vi "Initialize_GL.vi"(0 "Motion Settings":T1={"No Motion?"=FALSE, "Motion System"=enum."NI 735x", "Motion Bd ID"=1, "Motion Profile"="SMAC1", "# Axis"=1, "Reverse Z axis?"=TRUE, "SMAC Axis"=0, "scan pair"=enum."y-(x) scan", "RT fps"=6.0, "Steps per mm"=[1000, 1000, 1000, 1000], "Motor Parameters"={"velocity ct/s"=[10000.0, 10000.0, 10000.0, 50000.0], "accel ct/s^2"=[50000.0, 50000.0, 50000.0, 200000.0]}, "One Way Scan"=FALSE, "Reverse One Way Scan"=FALSE, "Global Position (mm)"=[], "Plane"=0, "Distance between\nscan lines (um)"=0.0, "Distance between\nscan planes (um)"=0.0, "number of scan planes"=1, "Total steps in line"=0, "Xtra plane\ndistance  (um)"=100, "Xtra planes "=1, "Add Axis"=FALSE, "overshoot cts"=200, "BKPT Shift"=0, "Scan Start Time (ms)"=0, "ESP VISA"="GPIB::1::INSTR", "3rd Axis"=1, "GL Ref Out"=refnum, "Galil Address"=""} {"3rd Axis" items=["x", "y", "z", "w"]; "Xtra planes" min=1; "Xtra plane\ndistance  (um)" min=0; "Distance between\nscan planes (um)" format="%.2f"; "Distance between\nscan lines (um)" format="%.2f"; "SMAC Axis" items=["None"=0, "Axis 1"=1, "Axis 2"=2, "Axis 3"=3, "Axis 4"=4, "Axis 5"=5, "Axis 6"=6, "Axis 7"=7, "Axis 8"=8, "Vector Space 1"=17, "Vector Space 2"=18, "Vector Space 3"=19, "Vector Space 4"=20]; "Motion Bd ID" min=1 max=32 step=1}, 2 "Location":T5, 3 "error in":errorcluster) -> (5 "Motion Settings":T1={"No Motion?"=FALSE, "Motion System"=enum."NI 735x", "Motion Bd ID"=1, "Motion Profile"="SMAC1", "# Axis"=1, "Reverse Z axis?"=TRUE, "SMAC Axis"=0, "scan pair"=enum."y-(x) scan", "RT fps"=6.0, "Steps per mm"=[1000, 1000, 1000, 1000], "Motor Parameters"={"velocity ct/s"=[10000.0, 10000.0, 10000.0, 50000.0], "accel ct/s^2"=[50000.0, 50000.0, 50000.0, 200000.0]}, "One Way Scan"=FALSE, "Reverse One Way Scan"=FALSE, "Global Position (mm)"=[], "Plane"=0, "Distance between\nscan lines (um)"=0.0, "Distance between\nscan planes (um)"=0.0, "number of scan planes"=1, "Total steps in line"=0, "Xtra plane\ndistance  (um)"=100, "Xtra planes "=1, "Add Axis"=FALSE, "overshoot cts"=200, "BKPT Shift"=0, "Scan Start Time (ms)"=0, "ESP VISA"="GPIB::1::INSTR", "3rd Axis"=1, "GL Ref Out"=refnum, "Galil Address"=""} {"3rd Axis" items=["x", "y", "z", "w"]; "Xtra planes" min=1; "Xtra plane\ndistance  (um)" min=0; "Distance between\nscan planes (um)" format="%.2f"; "Distance between\nscan lines (um)" format="%.2f"; "SMAC Axis" items=["None"=0, "Axis 1"=1, "Axis 2"=2, "Axis 3"=3, "Axis 4"=4, "Axis 5"=5, "Axis 6"=6, "Axis 7"=7, "Axis 8"=8, "Vector Space 1"=17, "Vector Space 2"=18, "Vector Space 3"=19, "Vector Space 4"=20]; "Motion Bd ID" min=1 max=32 step=1}, 6 "Initialization Failed!!":bool, 7 "error out":errorcluster)   [LabVIEW 2022 SP3]
uses:
  NI_controller/-NI_MotionRoutines/MotionParameters.ctl
  NI_controller/-NI_MotionRoutines/MotionSys.ctl
  -MotionRoutines/ScanAxis.ctl
  -MotionRoutines/3rdAxis.ctl
  -ScanSystem/Controls/location.ctl
  Command Menu.ctl
  GL Axis Control.ctl
panel:
  # "1-D and 2-D B scan settings"
  # "1-D and 2-D B scan settings"
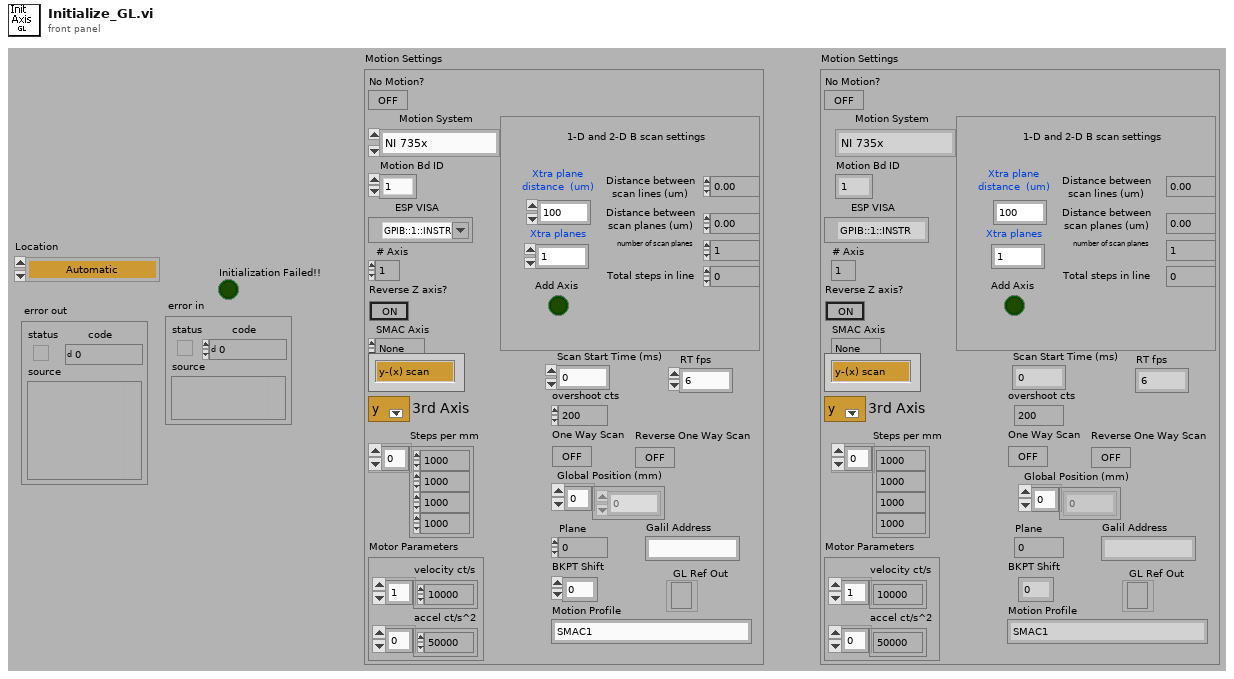
[diagram p1: front panel]
types:
  T1 = typedef "MotionParameters.ctl" = cluster{"No Motion?":bool, "Motion System":T2, "Motion Bd ID":u8, "Motion Profile":string, "# Axis":i8, "Reverse Z axis?":bool, "SMAC Axis":u16, "scan pair":T3, "RT fps":sgl, "Steps per mm":i32[], "Motor Parameters":cluster{"velocity ct/s":dbl[], "accel ct/s^2":dbl[]}, "One Way Scan":bool, "Reverse One Way Scan":bool, "Global Position (mm)":dbl[], "Plane":i32, "Distance between\nscan lines (um)":sgl, "Distance between\nscan planes (um)":sgl, "number of scan planes":i32, "Total steps in line":i32, "Xtra plane\ndistance  (um)":i32, "Xtra planes ":i32, "Add Axis":bool, "overshoot cts":i32, "BKPT Shift":i32, "Scan Start Time (ms)":u32, "ESP VISA":refnum<visa-resource-name>, "3rd Axis":T4, "GL Ref Out":refnum<k7>, "Galil Address":string}
  T2 = typedef "MotionSys.ctl" = enum16{"MM3000", "NI 735x", "Newport ESP", "No Motion Card", "Galil"}
  T3 = typedef "ScanAxis.ctl" = enum16{"y-(x) scan", "x-(y) scan", "z-(x) scan", "z-(y) scan", "y-(z) scan", "x-(z) scan", "w-(x) scan", "w-(y) scan", "w-(z) scan", "x-(w) scan", "y-(w) scan", "z-(w) scan"}
  T4 = typedef "3rdAxis.ctl" = u16
  T5 = typedef "location.ctl" = enum16{"Automatic", "WCM Main", "Hawaii", "Columbia MM3000", "Columbia  NI System", "NYU", "RRI 2", "UHI Allen", "CUMC RT", "Chiba", "Stony Brook", "WCM Microscopy", "WCM Aeoretch", "WCM Optics Lab", "WCM Main 2Axis", "WCM Rotation", "WCM SAM SMAC", "SERI GP", "SERI SAM 2023"}
  T6 = enum16{"Left Button", "Center Button", "Right Button", "Window Close"}
  T7 = typedef "Command Menu.ctl" = enum16{"CommandPassThrough", "Abort Motion", "Define Pos", "Velocity", "Acceleration", "Deceleration", "Position Rel", "Postion Abs", "Begin Move", "After Move", "Home", "KI", "KD", "KP", "IL", "Config I/O", "Set Bit", "Clear Bit", "Motor Off", "Moto On", "Status", "Execute", "Halt Execute", "HX Status", "Tell Velocity", "Check Motion", "BreakPoint", "Tell Position", "Current Code Line", "Tell Switches", "OC Force On", "OC Off", "Pos Soft Limit", "Rev Soft Limit"}
  T8 = cluster{"KD":i32, "KI":dbl, "KP":i32, "IL":i32}[]
  T9 = cluster{"KD":i32, "KI":i32, "KP":i32, "IL":i32}[]
  T10 = typedef "GL Axis Control.ctl" = u16
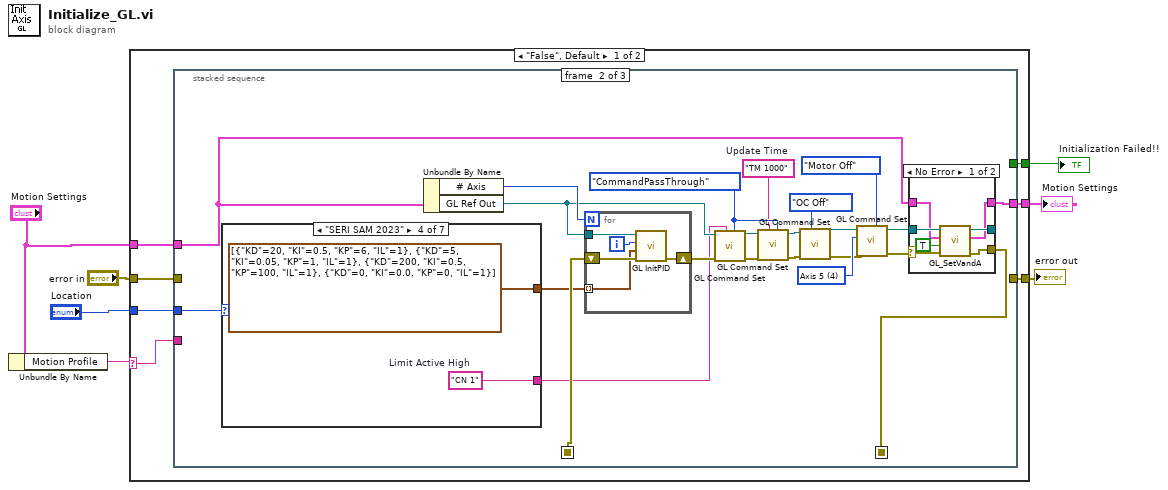
[diagram p0: block diagram]
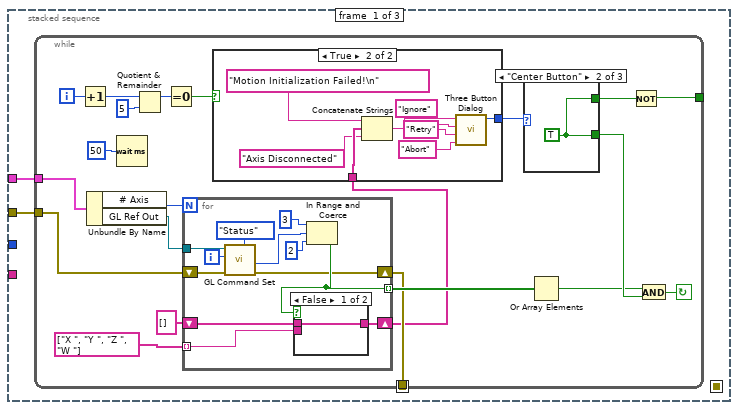
[diagram p2: hidden frame]
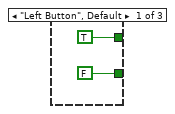
[diagram p3: hidden frame]
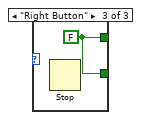
[diagram p4: hidden frame]
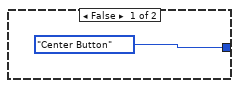
[diagram p5: hidden frame]
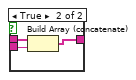
[diagram p6: hidden frame]
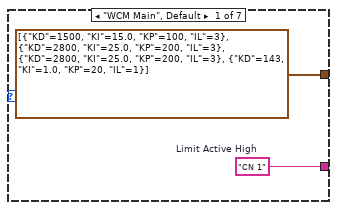
[diagram p8: hidden frame]
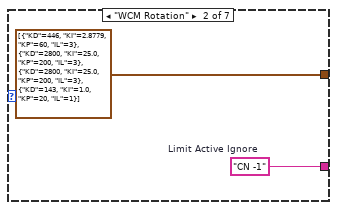
[diagram p9: hidden frame]
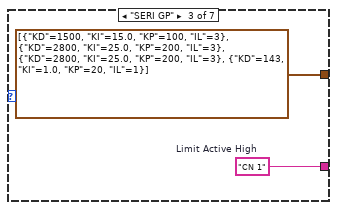
[diagram p10: hidden frame]
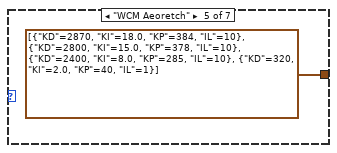
[diagram p11: hidden frame]
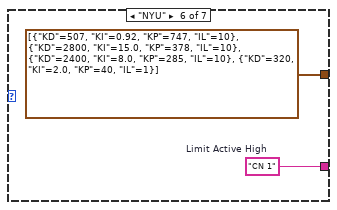
[diagram p12: hidden frame]
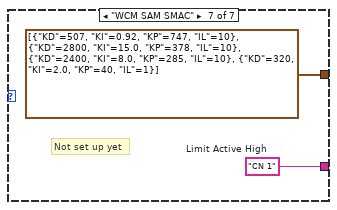
[diagram p13: hidden frame]
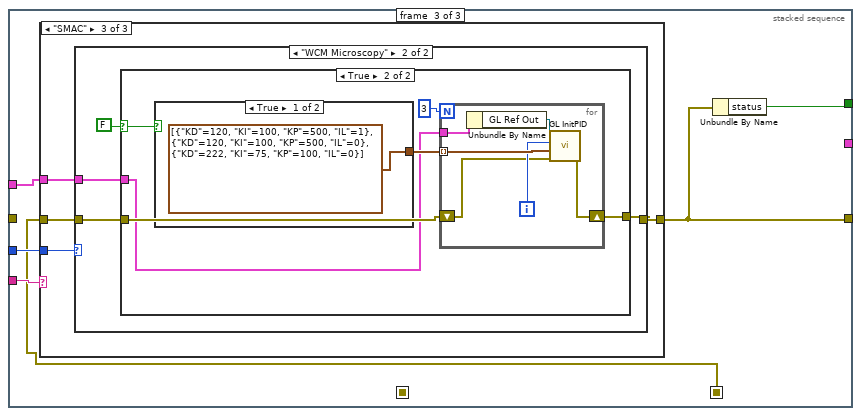
[diagram p14: hidden frame]
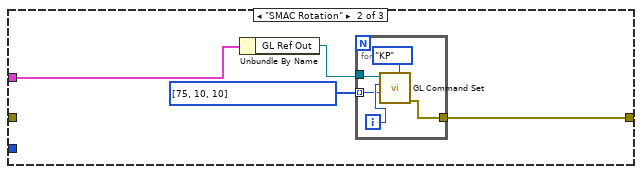
[diagram p16: hidden frame]
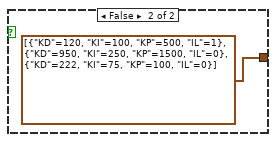
[diagram p19: hidden frame]
diagram:
  n1 = Unbundle By Name("Motion Settings") -> ("Motion Profile"=w4:string)
  n2 = case shown="\"False\", Default" w4 {
    selector: w4 -> [w11 _]
    tunnel: [w14 w160] -> w5
    tunnel: "Motion Settings" -> [w13 w159]
    tunnel: "error in" -> [w9 w160]
    tunnel: [w12 _] -> w6
    tunnel: "Location" -> [w10 _]
    tunnel: [w8 w159] -> w1
    frame "False", Default {
      n3 = stacked-sequence {
        seq-local: [w16 _ _] -> [_ w89 _]
        seq-local: [_ w69 _] -> [_ _ w121]
        tunnel: [_ _ w119] -> w14
        tunnel: w13 -> [w17 w87 w122]
        tunnel: w9 -> [w15 _ _]
        tunnel: [_ _ w120] -> w12
        tunnel: w11 -> [_ _ w124]
        tunnel: w10 -> [_ w68 w123]
        tunnel: [_ w70 _] -> w8
        frame #0 {
          n4 = while {
            tunnel: [w32] -> _
            tunnel: w17 -> [w25]
            tunnel: [w20] -> w16
            tunnel: w15 -> [w19]
            i -> [w36]
            stop <- w33 continue-if-true
            n5 = Increment(x=w36) -> (x+1=w34:i32)
            n6 = Unbundle By Name(w25) -> ("# Axis"=w30:i8, "GL Ref Out"=w21:refnum<k7>)
            n7 = Wait (ms)(milliseconds to wait=u32 50) -> ()  [unwired: 1 out]
            n8 = Quotient & Remainder(x=w34, y=5 ("x")) -> (x-y*floor(x/y)=w37:i32)  [unwired: 1 out]
            n9 = Equal To 0?(x=w37) -> (x = 0?=w38:bool)
            n10 = for {
              N: w30 -> [_]
              shift-right: [w63] -> w18
              shift-left: string[] [] -> [w62]
              tunnel: string[] ["X ", "Y ", "Z ", "W "] -> [w52] mode=indexing
              tunnel: w21 -> [w60]
              tunnel: [w55] -> w24 mode=indexing
              shift-right: [w53] -> w20
              shift-left: w19 -> [w54]
              i -> [w56]
              n11 = call "GL Command Set.vi"("Command"=Command_Menu."Status", "error in (no error)"=w54, "Axis"=w56, "Galil.IGalil"=w60) -> ("error out"=w53:errorcluster, "Response#"=w57:i32)  [unwired: 3 in, 3 out]
              n12 = In Range and Coerce(upper limit=3, x=w57, lower limit=2) -> (In Range?=w55:bool)  [unwired: 1 out]
              n13 = case shown="False" w55 {
                tunnel: [w64 w66] -> w63
                tunnel: w62 -> [w64 w67]
                tunnel: w52 -> [_ w65]
                frame False {
                }
                frame True {
                  n14 = Build Array (concatenate)(w67, w65) -> (w66:string[])
                }
              }
            }
            n15 = case shown="True" w38 {
              tunnel: w18 -> [_ w48]
              tunnel: [T6."Center Button" ("Which Button?") w46] -> w22
              frame False {
              }
              frame True {
                n16 = Concatenate Strings("Motion Initialization Failed!\n" ("message"), w48, "Axis Disconnected" ("string")) -> (w49:string)
                n17 = call <vilib>:"Three Button Dialog.vi"("Right Button Text (\"Cancel\")"="Abort" ("F button name (\"Cancel\")"), "Center Button Text (\"No\")"="Retry" ("T button name (\"OK\")"), "Left Button Text (\"Yes\")"="Ignore" ("Right Button Text (\"Cancel\")"), "message"=w49) -> ("Which Button?"=w46:T6)  [unwired: 7 in]
              }
            }
            n18 = case shown="\"Center Button\"" w22 {
              tunnel: [FALSE w41 w42] -> w27
              tunnel: [TRUE w41 w42] -> w26
              frame "Left Button", Default {
              }
              frame "Center Button" {
                w41 = TRUE
              }
              frame "Right Button" {
                w42 = FALSE
                n19 = Stop() -> ()  [unwired: 1 in]
              }
            }
            n20 = Or Array Elements(Boolean array=w24) -> (logical OR=w23:bool)
            n21 = Not(x=w26) -> (.not. x?=w32:bool)
            n22 = And(x=w23, y=w27) -> (x .and. y?=w33:bool)
          }
        }
        frame #1 {
          w76 = "TM 1000"  # Update Time
          w82 = T10 4 items=["Axis 1", "Axis 2", "Axis 3", "Axis 4", "Axis 5", "Axis 6", "Axis 7", "Axis 8"] ("Axis")
          w77 = Command_Menu."CommandPassThrough" ("Command")
          n23 = case shown="\"SERI SAM 2023\"" w68 {
            tunnel: [T8 [{"KD"=1500, "KI"=15.0, "KP"=100, "IL"=3}, {"KD"=2800, "KI"=25.0, "KP"=200, "IL"=3}, {"KD"=2800, "KI"=25.0, "KP"=200, "IL"=3}, {"KD"=143, "KI"=1.0, "KP"=20, "IL"=1}] T8 [{"KD"=446, "KI"=2.8779, "KP"=60, "IL"=3}, {"KD"=2800, "KI"=25.0, "KP"=200, "IL"=3}, {"KD"=2800, "KI"=25.0, "KP"=200, "IL"=3}, {"KD"=143, "KI"=1.0, "KP"=20, "IL"=1}] T8 [{"KD"=1500, "KI"=15.0, "KP"=100, "IL"=3}, {"KD"=2800, "KI"=25.0, "KP"=200, "IL"=3}, {"KD"=2800, "KI"=25.0, "KP"=200, "IL"=3}, {"KD"=143, "KI"=1.0, "KP"=20, "IL"=1}] T8 [{"KD"=20, "KI"=0.5, "KP"=6, "IL"=1}, {"KD"=5, "KI"=0.05, "KP"=1, "IL"=1}, {"KD"=200, "KI"=0.5, "KP"=100, "IL"=1}, {"KD"=0, "KI"=0.0, "KP"=0, "IL"=1}] T8 [{"KD"=2870, "KI"=18.0, "KP"=384, "IL"=10}, {"KD"=2800, "KI"=15.0, "KP"=378, "IL"=10}, {"KD"=2400, "KI"=8.0, "KP"=285, "IL"=10}, {"KD"=320, "KI"=2.0, "KP"=40, "IL"=1}] T8 [{"KD"=507, "KI"=0.92, "KP"=747, "IL"=10}, {"KD"=2800, "KI"=15.0, "KP"=378, "IL"=10}, {"KD"=2400, "KI"=8.0, "KP"=285, "IL"=10}, {"KD"=320, "KI"=2.0, "KP"=40, "IL"=1}] T8 [{"KD"=507, "KI"=0.92, "KP"=747, "IL"=10}, {"KD"=2800, "KI"=15.0, "KP"=378, "IL"=10}, {"KD"=2400, "KI"=8.0, "KP"=285, "IL"=10}, {"KD"=320, "KI"=2.0, "KP"=40, "IL"=1}]] -> w88
            tunnel: [w106 w108 w110 w112 _ w115 w117] -> w83
            frame "WCM Main", Default {
              w106 = "CN 1"  # Limit Active High
            }
            frame "WCM Rotation" {
              w108 = "CN -1"  # Limit Active Ignore
            }
            frame "SERI GP" {
              w110 = "CN 1"  # Limit Active High
            }
            frame "SERI SAM 2023" {
              w112 = "CN 1"  # Limit Active High
            }
            frame "WCM Aeoretch" {
            }
            frame "NYU" {
              w115 = "CN 1"  # Limit Active High
            }
            frame "WCM SAM SMAC" {
              w117 = "CN 1"  # Limit Active High
              # "Not set up yet"
            }
          }
          n24 = Unbundle By Name(w87) -> ("# Axis"=w90:i8, "GL Ref Out"=w85:refnum<k7>)
          n25 = for {
            N: w90 -> [_]
            tunnel: w85 -> [w104]
            shift-right: [w103] -> w84
            shift-left: w89 -> [w102]
            tunnel: w88 -> [w101] mode=indexing
            i -> [w105]
            n26 = call "GL InitPID.vi"("error in"=w102, "ControPrams"=w101, "Axis"=w105, "Galil.IGalil"=w104) -> ("error out"=w103:errorcluster)  [unwired: 3 in, 2 out]
          }
          n27 = call "GL Command Set.vi"("Command"=w77, "Text Input"=w83, "error in (no error)"=w84, "Galil.IGalil"=w85) -> ("error out"=w78:errorcluster, "ref out"=w79:refnum<k7>)  [unwired: 3 in, 3 out]
          n28 = call "GL Command Set.vi"("Command"=w77, "Text Input"=w76, "error in (no error)"=w78, "Galil.IGalil"=w79) -> ("error out"=w74:errorcluster, "ref out"=w75:refnum<k7>)  [unwired: 3 in, 3 out]
          n29 = call "GL Command Set.vi"("Command"=Command_Menu."OC Off", "error in (no error)"=w74, "Galil.IGalil"=w75) -> ("error out"=w73:errorcluster, "ref out"=w80:refnum<k7>)  [unwired: 4 in, 3 out]
          n30 = call "GL Command Set.vi"("Command"=Command_Menu."Motor Off", "error in (no error)"=w73, "Axis"=w82, "Galil.IGalil"=w80) -> ("error out"=w71:errorcluster, "ref out"=w72:refnum<k7>)  [unwired: 3 in, 3 out]
          n31 = case shown="No Error" w71 {
            selector: w71 -> [w94 w98]
            tunnel: w87 -> [w93 w99]
            tunnel: [w97 w100] -> _
            tunnel: [w96 w99] -> w70
            tunnel: w72 -> [w95 w100]
            tunnel: [w92 w98] -> w69
            frame No Error {
              n32 = call "GL_SetVandA.vi"("error in"=w94, "ByPass Pop up?"=TRUE, "Motion Settings"=w93, "Refnum in"=w95) -> ("error out"=w92:errorcluster, "Motion Settings Out"=w96:T1, "ref out"=w97:refnum<k7>)  [unwired: 5 in]
            }
            frame Error {
            }
          }
        }
        frame #2 {
          n33 = case shown="\"SMAC\"" w124 {
            tunnel: w121 -> [w125 _ w138]
            tunnel: [w125 w127 w137] -> w119
            tunnel: w123 -> [_ _ w136]
            tunnel: w122 -> [_ w126 w135]
            frame "False", Default {
            }
            frame "SMAC Rotation" {
              n34 = Unbundle By Name(w126) -> ("GL Ref Out"=w128:refnum<k7>)
              n35 = for {
                tunnel: w128 -> [w133]
                tunnel: i32[] [75, 10, 10] -> [w131] mode=indexing
                tunnel: [w130] -> w127
                i -> [w132]
                n36 = call "GL Command Set.vi"("Command"=Command_Menu."KP", "Value"=w131, "Axis"=w132, "Galil.IGalil"=w133) -> ("error out"=w130:errorcluster)  [unwired: 3 in, 4 out]
              }
            }
            frame "SMAC" {
              n37 = case shown="\"WCM Microscopy\"" w136 {
                tunnel: w138 -> [w139 w143]
                tunnel: [w139 w142] -> w137
                tunnel: w135 -> [_ w140]
                frame "Automatic", Default {
                }
                frame "WCM Microscopy" {
                  n38 = case shown="True" FALSE {
                    selector: FALSE -> [_ w147]
                    tunnel: w143 -> [w144 w149]
                    tunnel: [w144 w148] -> w142
                    tunnel: w140 -> [_ w145]
                    frame False {
                    }
                    frame True {
                      n39 = case shown="True" w147 {
                        tunnel: [T9 [{"KD"=120, "KI"=100, "KP"=500, "IL"=1}, {"KD"=120, "KI"=100, "KP"=500, "IL"=0}, {"KD"=222, "KI"=75, "KP"=100, "IL"=0}] T9 [{"KD"=120, "KI"=100, "KP"=500, "IL"=1}, {"KD"=950, "KI"=250, "KP"=1500, "IL"=0}, {"KD"=222, "KI"=75, "KP"=100, "IL"=0}]] -> w150
                        frame True {
                        }
                        frame False {
                        }
                      }
                      n40 = for {
                        N: 3 -> [_]
                        tunnel: w150 -> [w158] mode=indexing
                        shift-right: [w154] -> w148
                        shift-left: w149 -> [w156]
                        tunnel: w145 -> [w153]
                        i -> [w157]
                        n41 = Unbundle By Name(w153) -> ("GL Ref Out"=w155:refnum<k7>)
                        n42 = call "GL InitPID.vi"("error in"=w156, "ControPrams"=w158, "Axis"=w157, "Galil.IGalil"=w155) -> ("error out"=w154:errorcluster)  [unwired: 3 in, 2 out]
                      }
                    }
                  }
                }
              }
            }
          }
          n43 = Unbundle By Name(w119) -> ("status"=w120:bool)
        }
      }
    }
    frame "XY_Stage" {
    }
  }
  "error out" <- w5
  "Initialization Failed!!" <- w6
  "Motion Settings" <- w1
